vi "Main.vi"() -> ()   [LabVIEW 2013]
uses:
  Controls/States.ctl
  Controls/CSVFGVStates.ctl
panel:
  in  "Checked In?":bool
  out "Student ID":i32
  out "Checked in":string
  out "Check -in Time":timestamp
  in  "Check In":bool
  in  "Student List":i32(listbox)
  in  "Quit":bool
  out "Cat Points":dbl
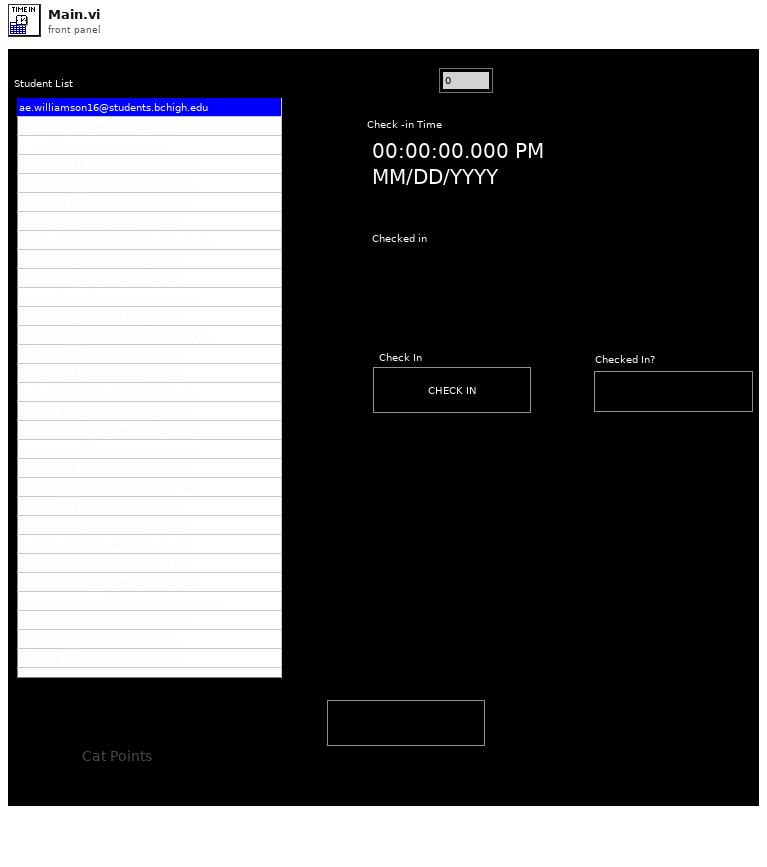
[diagram p1: front panel]
types:
  T1 = typedef "States.ctl" = enum16{"Init", "Idle", "Check In", "Quit"}
  T2 = typedef "CSVFGVStates.ctl" = enum16{"Init", "Read CSV", "Write CSV"}
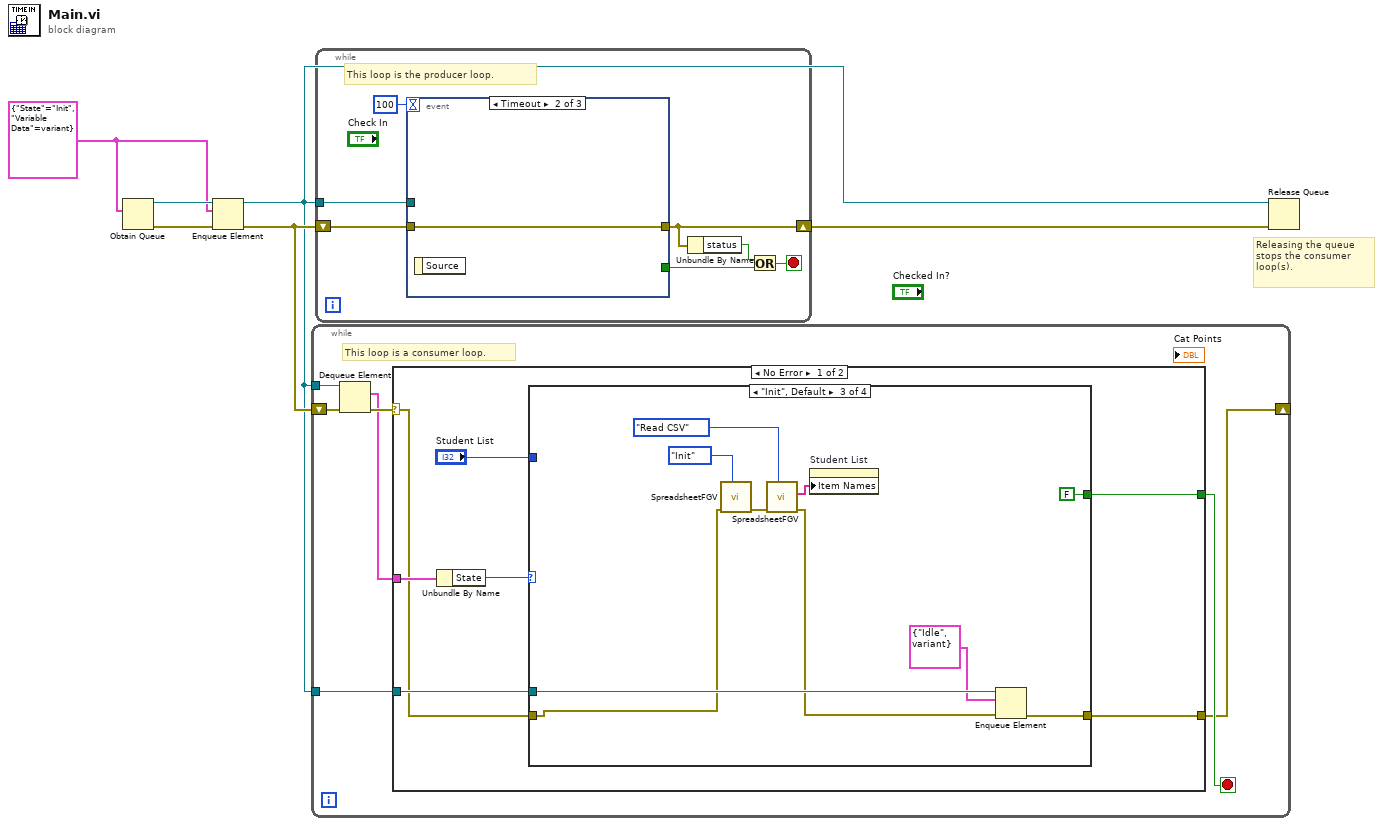
[diagram p0: block diagram]
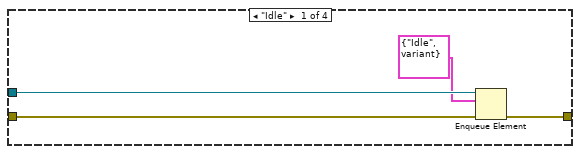
[diagram p2: hidden frame]
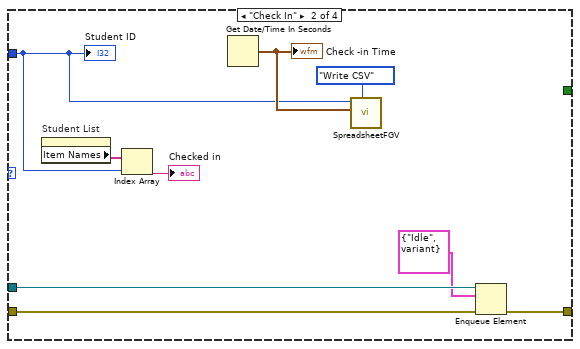
[diagram p3: hidden frame]
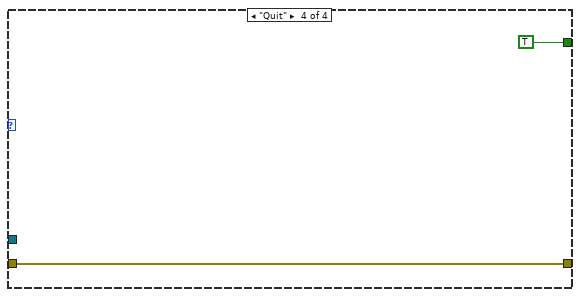
[diagram p4: hidden frame]
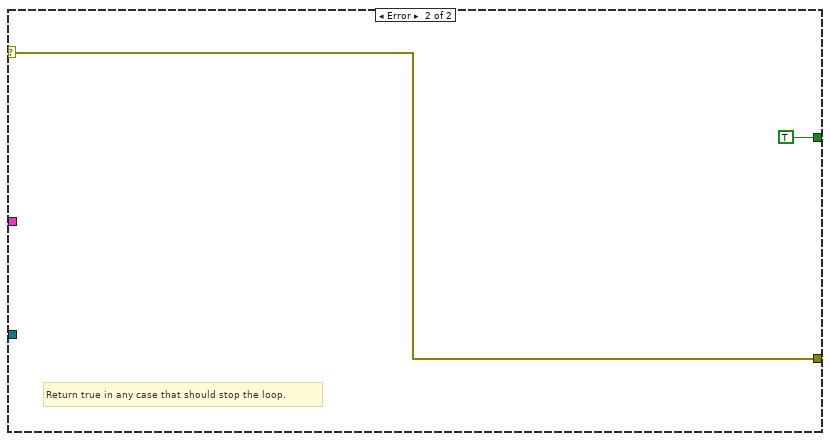
[diagram p5: hidden frame]
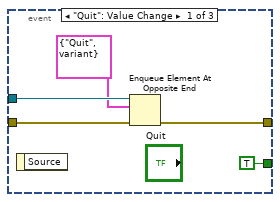
[diagram p6: hidden frame]
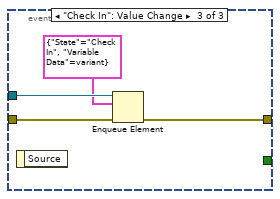
[diagram p7: hidden frame]
diagram:
  w4 = cluster{"State":T1, "Variable Data":variant} {"State"=enum."Init", "Variable Data"=variant}
  # "Releasing the queue stops the consumer loop(s)."
  n1 = Obtain Queue(element data type=w4) -> (queue out=w5:refnum<queue>, error out=w3:errorcluster)  [unwired: 4 in, 1 out]
  n2 = Enqueue Element(queue=w5, element=w4, error in (no error)=w3) -> (queue out=w1:refnum<queue>, error out=w2:errorcluster)  [unwired: 1 in, 1 out]
  n3 = while {
    tunnel: w1 -> [w13]
    tunnel: w1 -> [w8]
    shift-right: [w7] -> _
    shift-left: w2 -> [w10]
    stop <- w11 stop-if-true
    # "This loop is a consumer loop."
    n4 = Dequeue Element(queue=w13, error in (no error)=w10) -> (element=w9:cluster{"State":T1, "Variable Data":variant}, error out=w12:errorcluster)  [unwired: 1 in, 2 out]
    n5 = case shown="No Error" w12 {
      selector: w12 -> [w16 w46]
      tunnel: [w18 TRUE] -> w11
      tunnel: w9 -> [w20 _]
      tunnel: w8 -> [w17 _]
      tunnel: [w15 w46] -> w7
      frame No Error {
        n6 = Unbundle By Name(w20) -> ("State"=w19:T1)
        n7 = case shown="\"Init\", Default" w19 {
          tunnel: [_ _ FALSE ("Quit") TRUE ("Quit")] -> w18
          tunnel: w17 -> [w24 w33 w43 _]
          tunnel: w16 -> [w23 w32 w38 w44]
          tunnel: [w22 w31 w42 w44] -> w15
          tunnel: "Student List" -> [_ w26 _ _]
          frame "Idle" {
            n8 = Enqueue Element(queue=w24, element=cluster{"State":T1, "Variable Data":variant} {"State"=enum."Idle", "Variable Data"=variant}, error in (no error)=w23) -> (error out=w22:errorcluster)  [unwired: 1 in, 2 out]
          }
          frame "Check In" {
            n9 = property on="Student List" class="LstBox (strict)"() -> ("Item Names"=w29:string[])  [unwired: 2 in, 2 out]
            n10 = Index Array(array=w29, index=w26) -> (element=→"Checked in":string)
            n11 = Get Date/Time In Seconds() -> (seconds since 1Jan1904=w27:timestamp)
            "Check -in Time" <- w27
            n12 = call "SpreadsheetFGV.vi"("FGV Control"=CSVFGVStates."Write CSV", "Check -in Time"=w27, "Student ID"=w26) -> ()  [unwired: 7 in, 2 out]
            n13 = Enqueue Element(queue=w33, element=cluster{"State":T1, "Variable Data":variant} {"State"=enum."Idle", "Variable Data"=variant}, error in (no error)=w32) -> (error out=w31:errorcluster)  [unwired: 1 in, 2 out]
            "Student ID" <- w26
          }
          frame "Init", Default {
            n14 = call "SpreadsheetFGV.vi"("FGV Control"=CSVFGVStates."Init", "Error In"=w38) -> ("Error Out"=w37:errorcluster)  [unwired: 8 in, 1 out]
            n15 = call "SpreadsheetFGV.vi"("FGV Control"=CSVFGVStates."Read CSV", "Error In"=w37) -> ("Error Out"=w35:errorcluster, "Student Names"=w34:string[])  [unwired: 8 in]
            n16 = property on="Student List" class="LstBox (strict)"("Item Names"=w34) -> ()  [unwired: 2 in, 2 out]
            n17 = Enqueue Element(queue=w43, element=cluster{"State":T1, "Variable Data":variant} {"State"=enum."Idle", "Variable Data"=variant}, error in (no error)=w35) -> (error out=w42:errorcluster)  [unwired: 1 in, 2 out]
          }
          frame "Quit" {
          }
        }
      }
      frame Error {
        # "Return true in any case that should stop the loop."
      }
    }
  }
  n18 = while {
    shift-right: [w50] -> w6
    shift-left: w2 -> [w53]
    tunnel: w1 -> [w54]
    stop <- w51 stop-if-true
    # "This loop is the producer loop."
    n19 = event shown="[1] Timeout" {
      selector: _ -> [_ _ _]
      dyn-events: _ -> [_ _ _]
      timeout: 100 -> [_ _ _]
      tunnel: w54 -> [w56 _ w62]
      tunnel: w53 -> [w58 w60 w64]
      tunnel: [w57 w60 w63] -> w50
      tunnel: [TRUE ("Quit") _ _] -> w52
      event "Quit": Value Change {
        n20 = event-data() -> ()  [unwired: 1 in, 1 out]
        n21 = Enqueue Element At Opposite End(queue=w56, element=cluster{"Enum":T1, "variant":variant} {"Enum"=enum."Quit", "variant"=variant}, error in (no error)=w58) -> (error out=w57:errorcluster)  [unwired: 1 in, 2 out]
      }
      event Timeout {
        n22 = event-data() -> ()  [unwired: 1 in, 1 out]
      }
      event "Check In": Value Change {
        n23 = event-data() -> ()  [unwired: 1 in, 1 out]
        n24 = Enqueue Element(queue=w62, element=cluster{"State":T1, "Variable Data":variant} {"State"=enum."Check In", "Variable Data"=variant}, error in (no error)=w64) -> (error out=w63:errorcluster)  [unwired: 1 in, 2 out]
      }
    }
    n25 = Unbundle By Name(w50) -> ("status"=w49:bool)
    n26 = Or(x=w49, y=w52) -> (x .or. y?=w51:bool)
  }
  n27 = Release Queue(queue=w1, error in (no error)=w6) -> ()  [unwired: 1 in, 3 out]
